vi "Configure FFT Measurement Peak Search Markers.vi"(8 "error in (no error)":errorcluster, 9 "Number of Markers (1)":i32=1, 10 "Instance (1)":i32=1, 11 "VISA resource name":refnum<visa-resource-name>) -> (0 "error out":errorcluster, 3 "VISA resource name out":refnum<visa-resource-name>)   [LabVIEW 2020, in "Rohde&Schwarz CMXP GPRF.lvlib"]
doc: "Defines the number of active markers for the peak search.\n\nAttribute:\nRSCMXPGPRF_ATTR_FFT_MEASUREMENT_PEAK_SEARCH_MARKERS\n\nRemote-control command:\nCONFigure:GPRF:MEAS<i>:FFTSanalyzer:PSEarch:NOAMarkers"
uses:
  <instrlib>/Rohde&Schwarz CMXP GPRF/Rohde&Schwarz CMXP GPRF.lvlib
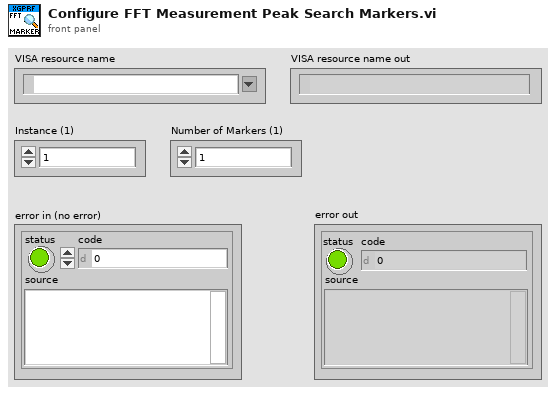
[diagram p1: front panel]
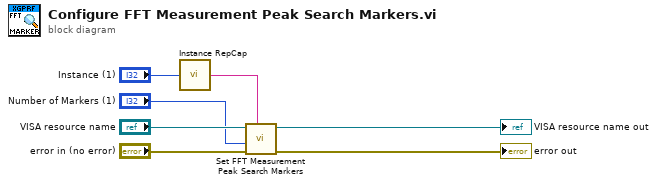
[diagram p0: block diagram]
diagram:
  n1 = call <instrlib>:"Instance RepCap.vi"("Instance in"="Instance (1)") -> ("Instance out"=w7:string)
  n2 = call "Set FFT Measurement Peak Search Markers"("Repeated Capabilities"=w7, "error in (no error)"="error in (no error)", "FFT Measurement Peak Search Markers (0)"="Number of Markers (1)", "instrument handle"="VISA resource name") -> ("error out"=→"error out":errorcluster, "instrument handle out"=→"VISA resource name out":refnum<visa-resource-name>)  [unwired: 6 in]
